vi "Get_Last_Error.vi"(8 "error in (no error)":errorcluster, 11 "mupExpr in":refnum<data-value>) -> (0 "error out":errorcluster, 2 "error details":T1, 3 "mupExpr out":refnum<data-value>)   [LabVIEW 2015, in "mupExpr.lvclass"]
doc: "Return the details of the last error that occured"
uses:
  mupExpr.lvclass
  mupExpr.lvclass/mupExpr.ctl
  mupLib/mupLibPath.vi
  mupLib/mupLib.lvlib
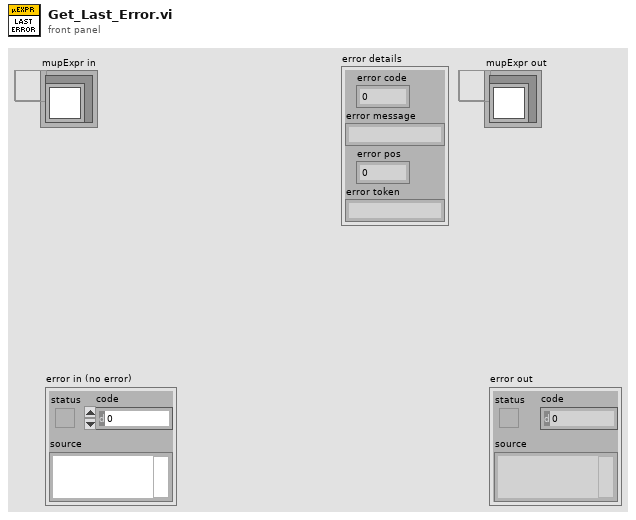
[diagram p1: front panel]
types:
  T1 = cluster{"error code":i32, "error message":string, "error pos":i32, "error token":string}
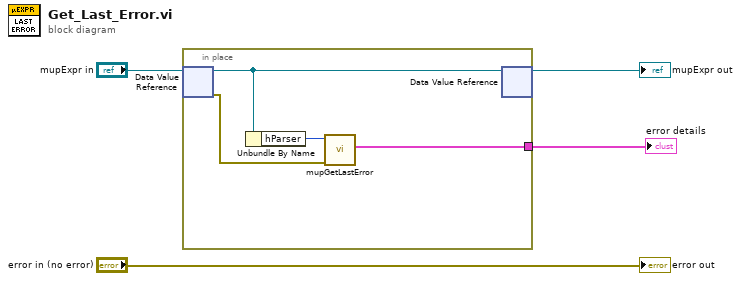
[diagram p0: block diagram]
diagram:
  n1 = in-place {
    in-place-border: [w5] -> w1
    n2 = in-place-dvr #1("mupExpr in") -> (w8:refnum<class "mupExpr.lvclass">, w6:errorcluster)
    n3 = Unbundle By Name(w8) -> ("hParser"=w7:u64)
    n4 = call "mupGetLastError.vi"("error in (no error)"=w6, "hParser in"=w7) -> ("error details"=w5:T1)  [unwired: 7 in, 2 out]
    n5 = in-place-dvr #1(w8) -> (→"mupExpr out":refnum<data-value>)  [unwired: 1 out]
  }
  "error details" <- w1
  "error out" <- "error in (no error)"
